vi "SVX Shaft Centerline Plot.vi"(0 "DC gaps":T5(array[cluster]) {"DC gap value" format="%.2f"; "time/rev/RPM" format="%.2f"}, 1 "unit labels":T1(array[cluster]), 2 "gap position info":T4, 5 "error in (no error)":errorcluster, 7 "channel properties":T2[](array[typedef]) {"probe angle [deg]" max=360; "direction" items=["CCW", "CW"]}, 8 "reset? (F)":bool) -> (14 "shaft centerline":T3(array[cluster]), 19 "error out":errorcluster)   [LabVIEW 2017, in "SoundVib_MCMDisplay.lvlib"]
doc: "Prepares shaft centerline plot data for displaying on a Shaft Centerline Plot. A shaft centerline plot displays the averaged positions of the shaft center. Use this VI to measure the movement of the shaft center over time."
uses:
  <vilib>/addons/Sound and Vibration/Order Analysis/Data Presentation/SoundVib_MCMDisplay.lvlib
  <vilib>/addons/Sound and Vibration/Order Analysis/Misc/OAT Position Info.ctl
  <vilib>/addons/Sound and Vibration/Order Analysis/Data Presentation/SubVIs/OAT MCM Channel Property.ctl
  <vilib>/addons/Sound and Vibration/Order Analysis/Misc/SVMS Attribute.ctl
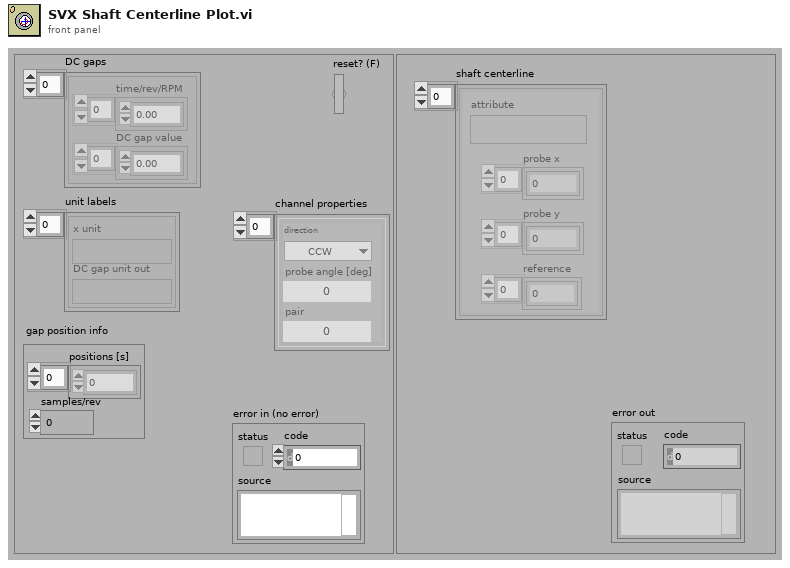
[diagram p1: front panel]
types:
  T1 = cluster{"x unit":string, "DC gap unit out":string}[]
  T2 = typedef "OAT MCM Channel Property.ctl" = cluster{"direction":u16, "probe angle [deg]":u16, "pair":u16}
  T3 = cluster{"probe x":dbl[], "probe y":dbl[], "reference":dbl[], "attribute":variant}[]
  T4 = typedef "OAT Position Info.ctl" = cluster{"positions [s]":dbl[], "samples/rev":dbl}
  T5 = cluster{"time/rev/RPM":dbl[], "DC gap value":dbl[]}[]
  T6 = cluster{"DC gap value X":dbl[], "DC gap value Y":dbl[], "reference":dbl[], "attribute":variant}
  T7 = typedef "SVMS Attribute.ctl" = u16
  T8 = cluster{"x unit":string, "DC gap unit out":string}
  T9 = cluster{"time/rev/RPM":dbl[], "DC gap value":dbl[]}
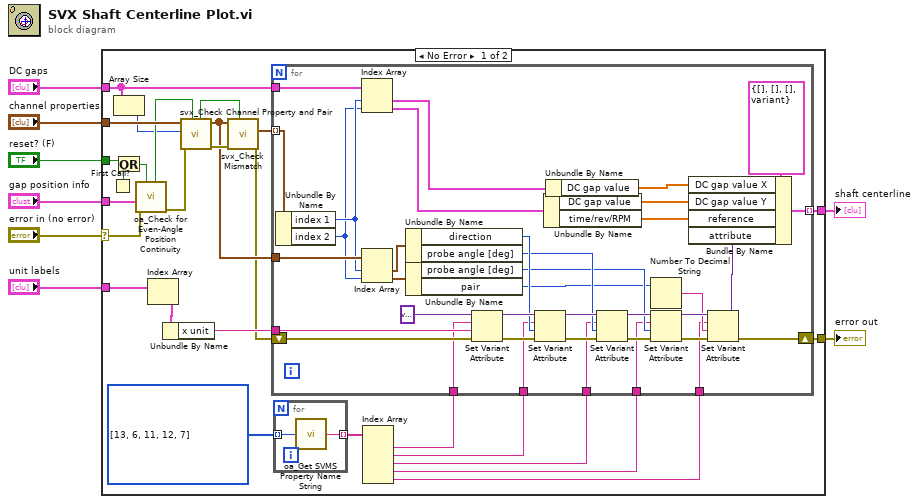
[diagram p0: block diagram]
diagram:
  n1 = case shown="No Error" "error in (no error)" {
    selector: "error in (no error)" -> [w31 w75]
    tunnel: "reset? (F)" -> [w33 _]
    tunnel: "gap position info" -> [w35 _]
    tunnel: "DC gaps" -> [w18 _]
    tunnel: "channel properties" -> [w26 _]
    tunnel: [w30 w75] -> w4
    tunnel: "unit labels" -> [w29 _]
    tunnel: [w17 _] -> w1
    frame No Error {
      w15 = T7[] [13, 6, 11, 12, 7] items=["Pulse / Revolution", "Slope", "Threshold", "Hysteresis", "Order", "Reference Label", "Rotation Direction", "Pair String", "Polar Plot Type", "Sample Per Revolution", "Probe Angle", "Probe Angle X", "Probe Angle Y", "X Axis Unit", "OTB Plot Type"]
      n2 = First Call?() -> (First Call?: T/F=w34:bool)
      n3 = Array Size(array=w18) -> (size(s)=w23:i32)
      n4 = Or(x=w33, y=w34) -> (x .or. y?=w32:bool)
      n5 = call <vilib>:"oa_Check for Even-Angle Position Continuity.vi"("reset in"=w32, "error in (no error)"=w31, "even-angle position info"=w35) -> ("error out"=w25:errorcluster, "position not continuous"=w24:bool)  [unwired: 6 in, 1 out]
      n6 = Index Array(array=w29) -> (element=w28:T8)  [unwired: 1 in]
      n7 = Unbundle By Name(w28) -> ("x unit"=w27:string)
      n8 = call <vilib>:"svx_Check Channel Property and Pair.vi"("reset in"=w24, "error in (no error)"=w25, "channel number"=w23, "channel property"=w26) -> ("error out"=w22:errorcluster, "channel property out"=w20:T2[], "reset out"=w21:bool)  [unwired: 5 in]
      n9 = call <vilib>:"svx_Check Mismatch.vi"("reset in"=w21, "error in (no error)"=w22, "channel property in"=w20) -> ("error out"=w19:errorcluster, "pair index"=w16:cluster{"index 1":i32, "index 2":i32}[])  [unwired: 5 in, 2 out]
      n10 = for {
        tunnel: w15 -> [w37] mode=indexing
        tunnel: [w36] -> w14 mode=indexing
        n11 = call <vilib>:"oa_Get SVMS Property Name String.vi"("attribute"=w37) -> ("attribute name"=w36:string)  [unwired: 4 in]
      }
      n12 = Index Array(array=w14) -> (element #1=w13:string, element #2=w12:string, element #3=w11:string, element #4=w10:string, element #5=w9:string)  [unwired: 5 in]
      n13 = for {
        tunnel: w27 -> [w74]
        shift-right: [w73] -> w30
        shift-left: w19 -> [w52]
        tunnel: w16 -> [w53] mode=indexing
        tunnel: w20 -> [w51]
        tunnel: w18 -> [w48]
        tunnel: [w43] -> w17 mode=indexing
        tunnel: w13 -> [w42]
        tunnel: w12 -> [w41]
        tunnel: w11 -> [w40]
        tunnel: w10 -> [w39]
        tunnel: w9 -> [w38]
        n14 = Unbundle By Name(w53) -> ("index 1"=w47:i32, "index 2"=w46:i32)
        n15 = Index Array(array=w48, index #1=w47, index #2=w46) -> (element #1=w44:T9, element #2=w45:T9)
        n16 = Index Array(array=w51, index #1=w47, index #2=w46) -> (element #1=w50:T2, element #2=w49:T2)
        n17 = Unbundle By Name(w50) -> ("direction"=w62:u16, "probe angle [deg]"=w61:u16)
        n18 = Unbundle By Name(w49) -> ("probe angle [deg]"=w60:u16, "pair"=w55:u16)
        n19 = Set Variant Attribute(Variant=variant ("variant"), name=w42, value=w74, error in=w52) -> (Variant out=w64:variant, error out=w65:errorcluster)  [unwired: 1 out]
        n20 = Set Variant Attribute(Variant=w64, name=w41, value=w62, error in=w65) -> (Variant out=w69:variant, error out=w68:errorcluster)  [unwired: 1 out]
        n21 = Unbundle By Name(w45) -> ("DC gap value"=w71:dbl[], "time/rev/RPM"=w70:dbl[])
        n22 = Unbundle By Name(w44) -> ("DC gap value"=w72:dbl[])
        n23 = Set Variant Attribute(Variant=w69, name=w40, value=w61, error in=w68) -> (Variant out=w66:variant, error out=w67:errorcluster)  [unwired: 1 out]
        n24 = Number To Decimal String(number=w55) -> (decimal integer string=w54:string)  [unwired: 1 in]
        n25 = Set Variant Attribute(Variant=w66, name=w39, value=w60, error in=w67) -> (Variant out=w59:variant, error out=w58:errorcluster)  [unwired: 1 out]
        n26 = Set Variant Attribute(Variant=w59, name=w38, value=w54, error in=w58) -> (Variant out=w57:variant, error out=w73:errorcluster)  [unwired: 1 out]
        n27 = Bundle By Name(cluster=T6 {"DC gap value X"=[], "DC gap value Y"=[], "reference"=[], "attribute"=variant} ("element"), "DC gap value X"=w72, "DC gap value Y"=w71, "reference"=w70, "attribute"=w57) -> (w43:T6)
      }
    }
    frame Error {
    }
  }
  "error out" <- w4
  "shaft centerline" <- w1
